vi "rs3 end processing.vi"(8 "error in (no error)":errorcluster, 10 "Processing Queues":T1, 11 "Processing Blocks":T2) -> (0 "error out":errorcluster)   [LabVIEW 2017, in "libRealSense3.lvlib"]
doc: "Clean up and close all post-processing block & queues"
uses:
  libRealSense3.lvlib
panel:
  # "RS3 End Post-Processing"
  # "(C) Intel Corp.,  AGJ"
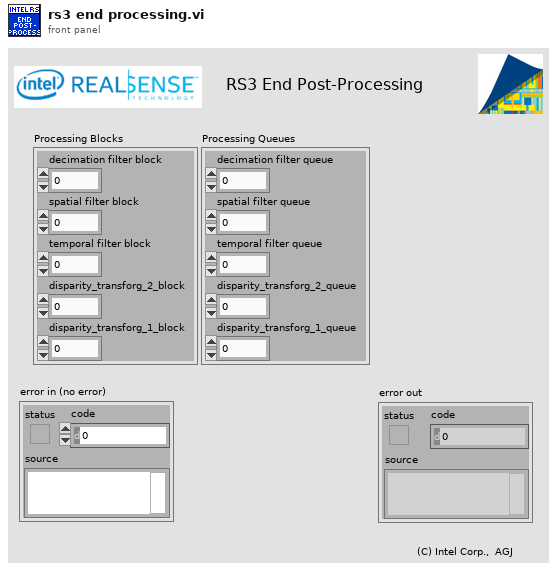
[diagram p1: front panel]
types:
  T1 = cluster{"decimation filter queue":u64, "spatial filter queue":u64, "temporal filter queue":u64, "disparity_transforg_2_queue":u64, "disparity_transforg_1_queue":u64}
  T2 = cluster{"decimation filter block":u64, "spatial filter block":u64, "temporal filter block":u64, "disparity_transforg_2_block":u64, "disparity_transforg_1_block":u64}
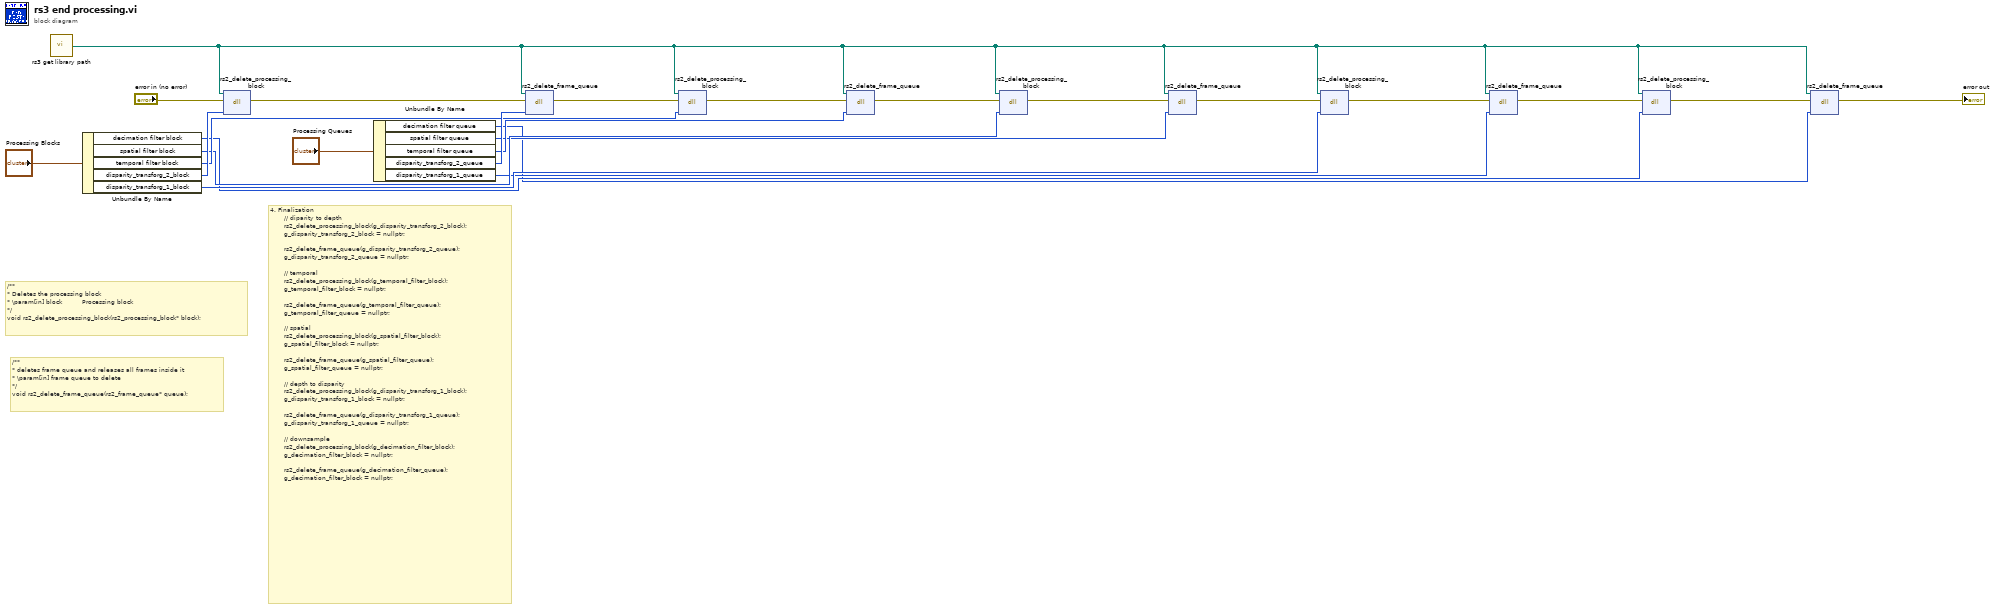
[diagram p0: block diagram]
diagram:
  # "/**\n* deletes frame queue and releases all frames inside it\n* \\param[in] frame queue to delete\n*/\nvoid rs2_delete_frame_queue(rs2_frame_queue* queue);"
  # "/**\n* Deletes the processing block\n* \\param[in] block          Processing block\n*/\nvoid rs2_delete_processing_block(rs2_processing_block* block);"
  # "4. Finalization\n       // diparity to depth\n       rs2_delete_processing_block(g_disparity_transforg_2_block);\n       g_disparity_transforg_2_block = nullptr;\n\n       rs2_delete_frame_queue(g_disparity_transforg_2_queue);\n       g_disparity_transforg_2_queue = nullptr;\n\n       // temporal\n       rs2_delete_processing_block(g_temporal_filter_block);\n       g_temporal_filter_block = nullptr;\n\n       rs2_delete_frame_queue(g_temporal_filter_queue);\n       g_temporal_filter_queue = nullptr;\n\n       // spatial\n       rs2_delete_processing_block(g_spatial_filter_block);\n       g_spatial_filter_block = nullptr;\n\n       rs2_delete_frame_queue(g_spatial_filter_queue);\n       g_spatial_filter_queue = nullptr;\n\n       // depth to disparity\n       rs2_delete_processing_block(g_disparity_transforg_1_block);\n       g_disparity_transforg_1_block = nullptr;\n\n       rs2_delete_frame_queue(g_disparity_transforg_1_queue);\n       g_disparity_transforg_1_queue = nullptr;\n\n       // downsample\n       rs2_delete_processing_block(g_decimation_filter_block);\n       g_decimation_filter_block = nullptr;\n\n       rs2_delete_frame_queue(g_decimation_filter_queue);\n       g_decimation_filter_block = nullptr;"
  n1 = call "rs3 get library path.vi"() -> ("Realsense 2 Library Path"=w1:path)
  n2 = Unbundle By Name("Processing Blocks") -> ("decimation filter block"=w3:u64, "spatial filter block"=w7:u64, "temporal filter block"=w9:u64, "disparity_transforg_2_block"=w11:u64, "disparity_transforg_1_block"=w5:u64)
  n3 = dll-call lib="C:/Users/agrunnet/Documents/libRealSense6/realsense2.dll" fn="rs2_delete_processing_block"(path in=w1, error in="error in (no error)", "processing block"=w11) -> (error out=w23:errorcluster)  [unwired: 3 in, 1 out]
  n4 = Unbundle By Name("Processing Queues") -> ("decimation filter queue"=w2:u64, "spatial filter queue"=w6:u64, "temporal filter queue"=w8:u64, "disparity_transforg_2_queue"=w10:u64, "disparity_transforg_1_queue"=w4:u64)
  n5 = dll-call lib="C:/Users/agrunnet/Documents/libRealSense6/realsense2.dll" fn="rs2_delete_frame_queue"(path in=w1, error in=w23, "processing block"=w10) -> (error out=w21:errorcluster)  [unwired: 3 in, 1 out]
  n6 = dll-call lib="C:/Users/agrunnet/Documents/libRealSense6/realsense2.dll" fn="rs2_delete_processing_block"(path in=w1, error in=w21, "processing block"=w9) -> (error out=w22:errorcluster)  [unwired: 3 in, 1 out]
  n7 = dll-call lib="C:/Users/agrunnet/Documents/libRealSense6/realsense2.dll" fn="rs2_delete_frame_queue"(path in=w1, error in=w22, "processing block"=w8) -> (error out=w19:errorcluster)  [unwired: 3 in, 1 out]
  n8 = dll-call lib="C:/Users/agrunnet/Documents/libRealSense6/realsense2.dll" fn="rs2_delete_processing_block"(path in=w1, error in=w19, "processing block"=w7) -> (error out=w20:errorcluster)  [unwired: 3 in, 1 out]
  n9 = dll-call lib="C:/Users/agrunnet/Documents/libRealSense6/realsense2.dll" fn="rs2_delete_frame_queue"(path in=w1, error in=w20, "processing block"=w6) -> (error out=w17:errorcluster)  [unwired: 3 in, 1 out]
  n10 = dll-call lib="C:/Users/agrunnet/Documents/libRealSense6/realsense2.dll" fn="rs2_delete_processing_block"(path in=w1, error in=w17, "processing block"=w5) -> (error out=w18:errorcluster)  [unwired: 3 in, 1 out]
  n11 = dll-call lib="C:/Users/agrunnet/Documents/libRealSense6/realsense2.dll" fn="rs2_delete_frame_queue"(path in=w1, error in=w18, "processing block"=w4) -> (error out=w15:errorcluster)  [unwired: 3 in, 1 out]
  n12 = dll-call lib="C:/Users/agrunnet/Documents/libRealSense6/realsense2.dll" fn="rs2_delete_processing_block"(path in=w1, error in=w15, "processing block"=w3) -> (error out=w16:errorcluster)  [unwired: 3 in, 1 out]
  n13 = dll-call lib="C:/Users/agrunnet/Documents/libRealSense6/realsense2.dll" fn="rs2_delete_frame_queue"(path in=w1, error in=w16, "processing block"=w2) -> (error out=→"error out":errorcluster)  [unwired: 3 in, 1 out]
